vi "ReallyComplicatedSonar (SubVI).vi"(11 "Activate Shoot":bool) -> ()   [LabVIEW 2017]
uses:
  <vilib>/Rock Robotics/WPI/Solenoid/WPI_SolenoidValue.ctl
  <vilib>/Rock Robotics/WPI/Utilities/WPI_GetSetVariantRefNum.vi
  <vilib>/Rock Robotics/WPI/RobotDrive/WPI_RobotDriveArcadeDrive_Standard(NoSaturation).vi
  <vilib>/Rock Robotics/WPI/Solenoid/WPI_SolenoidSetEnum.vi
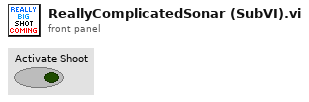
[diagram p1: front panel]
types:
  T1 = typedef "WPI_SolenoidValue.ctl" = enum16{"Off", "On", "Forward", "Reverse"}
  T2 = typedef "WPI_RobotDriveDevRef.ctl" = cluster{"DevStatus":errorcluster, "Motors[]":T3[], "Square Inputs":bool, "Max Output":dbl}
  T3 = typedef "WPI_MotorControlDeviceRef.ctl" = cluster{"DeviceStatus":errorcluster, "Type":T4, "PWM":cluster{"PWM Channel":T5, "DeadBand":T6}, "CAN":cluster{"Device Number":u8, "SetOutput VI Ref":variant, "GetOutput VI Ref":variant, "Enable VI Ref":variant, "Disable VI Ref":variant, "Data":variant}, "Invert":bool, "DIO PWM":cluster{"PWM \"Enable\" Channel":T5, "DIOChannel":T7, "PWM Rate":dbl}}
  T4 = typedef "WPI_MotorControlType.ctl" = enum16{"PWM", "CAN", "DIO PWM"}
  T5 = typedef "FPGA_DIOPWMChannel.ctl" = enum8{"PWM 0", "PWM 1", "PWM 2", "PWM 3", "PWM 4", "PWM 5", "PWM 6", "PWM 7", "PWM 8", "PWM 9", "PWM MXP 0", "PWM MXP 1", "PWM MXP 2", "PWM MXP 3", "PWM MXP 4", "PWM MXP 5", "PWM MXP 6", "PWM MXP 7", "PWM MXP 8", "PWM MXP 9", "Invalid"}
  T6 = typedef "WPI_PWMDeadband.ctl" = cluster{"Name":string, "maxPositivePwm":i32, "minPositivePwm":i32, "centerPwm":i32, "maxNegativePwm":i32, "minNegativePwm":i32, "angularRange":u16}
  T7 = typedef "FPGA_DIOChannel.ctl" = enum8{"DIO 0", "DIO 1", "DIO 2", "DIO 3", "DIO 4", "DIO 5", "DIO 6", "DIO 7", "DIO 8", "DIO 9", "DIO MXP 0", "DIO MXP 1", "DIO MXP 2", "DIO MXP 3", "DIO MXP 4", "DIO MXP 5", "DIO MXP 6", "DIO MXP 7", "DIO MXP 8", "DIO MXP 9", "DIO MXP 10", "DIO MXP 11", "DIO MXP 12", "DIO MXP 13", "DIO MXP 14", "DIO MXP 15", "SPI Port CS1", "SPI Port CS2", "SPI Port CS3", "SPI Port MISO", "SPI Port MOSI", "Invalid"}
  T8 = typedef "DriveMotors.ctl" = cluster{"MotorControlDevRef":T3, "MotorControlDevRef":T3, "MotorControlDevRef":T3, "MotorControlDevRef":T3, "MotorControlDevRef":T3, "MotorControlDevRef":T3}
  T9 = typedef "WPI_SolenoidDevRef.ctl" = cluster{"DevStatus":errorcluster, "Pneumatics Control Module":u8, "Forward Solenoid Channel":T10, "Reverse Solenoid Channel":T10}
  T10 = typedef "WPI_SolenoidChannel.ctl" = enum8{"Solenoid 0", "Solenoid 1", "Solenoid 2", "Solenoid 3", "Solenoid 4", "Solenoid 5", "Solenoid 6", "Solenoid 7", "Invalid"}
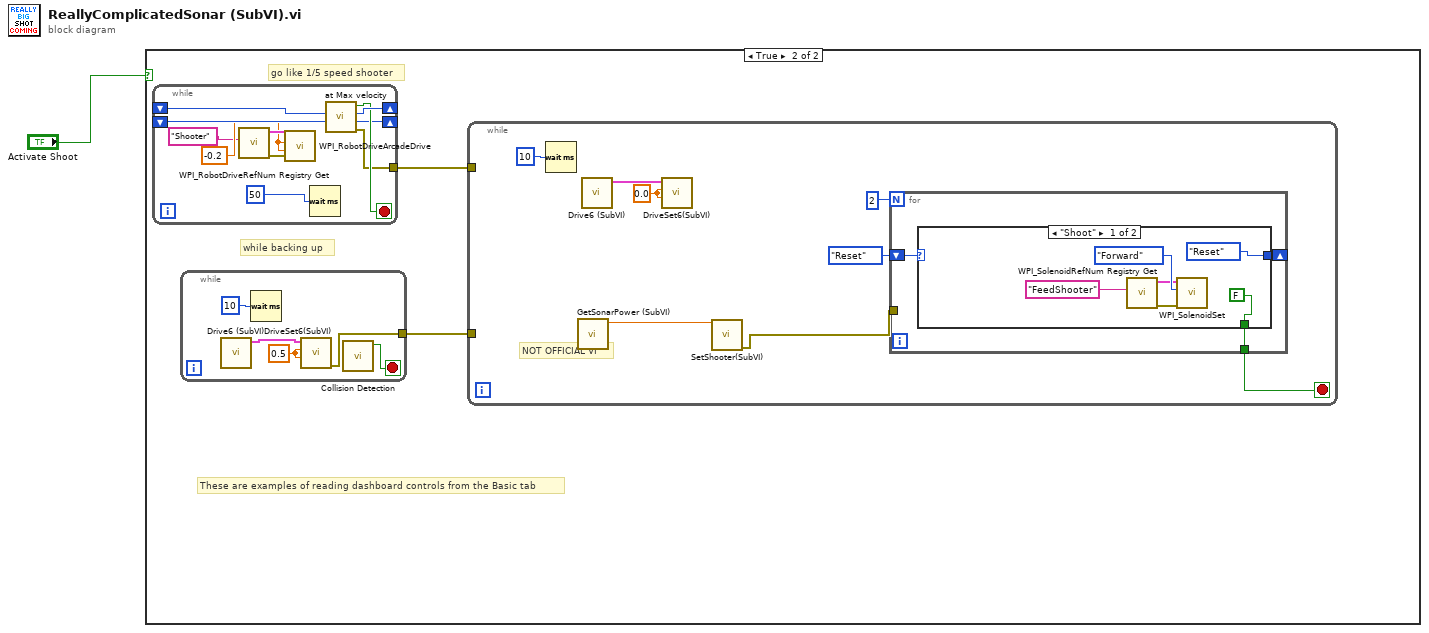
[diagram p0: block diagram]
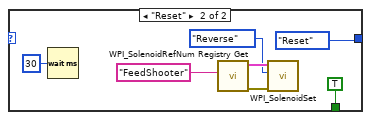
[diagram p3: hidden frame]
diagram:
  # "These are examples of reading dashboard controls from the Basic tab"
  n1 = case shown="True" "Activate Shoot" {
    frame False {
    }
    frame True {
      # "while backing up"
      # "go like 1/5 speed shooter"
      n2 = while {
        shift-right: [w40] -> _
        shift-left: _ -> [w42]
        shift-right: [w38] -> _
        shift-left: _ -> [w41]
        tunnel: [w37] -> w2
        stop <- w39 stop-if-true
        w34 = -0.2 ("Percentage")
        n3 = call <vilib>:"WPI_RobotDriveRefNum Registry Get.vi"("refnum name"="Shooter") -> ("error out"=w36:errorcluster, "RobotDriveDevRef"=w35:T2)  [unwired: 9 in]
        n4 = call-poly <vilib>:"WPI_RobotDriveArcadeDrive.vi"("error in (no error)"=w36, "Y axis value"=w34, "X axis value"=w34, "RobotDriveDevRef"=w35) -> ()  [unwired: 5 in, 3 out]
        n5 = Wait (ms)(milliseconds to wait=u32 50) -> ()  [unwired: 1 out]
        n6 = call "at Max velocity.vi"("Previous Velocity 2"=w41, "Previous Velocity"=w42) -> ("error out 2"=w37:errorcluster, "New Velocity 2"=w38:i32, "New Velocity"=w40:i32, "Max Velocity"=w39:bool)  [unwired: 6 in]
      }
      n7 = while {
        tunnel: [w28] -> w3
        stop <- w32 stop-if-true
        w29 = 0.5 ("Right")
        n8 = call "Drive6 (SubVI).vi"() -> ("DriveControlDevRef"=w30:T8)  [unwired: 10 in, 1 out]
        n9 = Wait (ms)(milliseconds to wait=u32 10) -> ()  [unwired: 1 out]
        n10 = call "DriveSet6(SubVI).vi"("Left"=w29, "Right"=w29, "output cluster"=w30) -> ("error out"=w28:errorcluster)  [unwired: 7 in, 1 out]
        n11 = call "Collision Detection.vi"() -> ("Colision Detected"=w32:bool)  [unwired: 11 in]
      }
      n12 = while {
        tunnel: w3 -> [_]
        tunnel: w2 -> [_]
        stop <- w5 stop-if-true
        w9 = 0.0 ("Right")
        # "NOT OFFICIAL VI"
        n13 = Wait (ms)(milliseconds to wait=u32 10) -> ()  [unwired: 1 out]
        n14 = call "GetSonarPower (SubVI).vi"() -> ("Value"=w8:dbl)  [unwired: 11 in]
        n15 = call "Drive6 (SubVI).vi"() -> ("DriveControlDevRef"=w10:T8)  [unwired: 10 in, 1 out]
        n16 = call "DriveSet6(SubVI).vi"("Left"=w9, "Right"=w9, "output cluster"=w10) -> ()  [unwired: 7 in, 2 out]
        n17 = call "SetShooter(SubVI).vi"("Velocity"=w8) -> ("error out"=w4:errorcluster)  [unwired: 10 in]
        n18 = for {
          N: 2 -> [_]
          shift-right: [w13] -> _
          shift-left: enum16{"Shoot", "Reset"}."Reset" -> [w14]
          tunnel: [w12] -> w5
          tunnel: w4 -> [_]
          n19 = case shown="\"Shoot\"" w14 {
            tunnel: [enum16{"Shoot", "Reset"}."Reset" enum16{"Shoot", "Reset"}."Reset"] -> w13
            tunnel: [FALSE TRUE] -> w12
            frame "Shoot" {
              n20 = call <vilib>:"WPI_SolenoidRefNum Registry Get.vi"("refnum name"="FeedShooter") -> ("error out"=w17:errorcluster, "SolenoidDevRef"=w18:T9)  [unwired: 9 in]
              n21 = call-poly <vilib>:"WPI_SolenoidSet.vi"("error in (no error)"=w17, "Value"=WPI_SolenoidValue."Forward", "SolenoidDevRef"=w18) -> ()  [unwired: 7 in, 2 out]
            }
            frame "Reset" {
              n22 = Wait (ms)(milliseconds to wait=u32 30) -> ()  [unwired: 1 out]
              n23 = call <vilib>:"WPI_SolenoidRefNum Registry Get.vi"("refnum name"="FeedShooter") -> ("error out"=w26:errorcluster, "SolenoidDevRef"=w27:T9)  [unwired: 9 in]
              n24 = call-poly <vilib>:"WPI_SolenoidSet.vi"("error in (no error)"=w26, "Value"=WPI_SolenoidValue."Reverse", "SolenoidDevRef"=w27) -> ()  [unwired: 7 in, 2 out]
            }
          }
        }
      }
    }
  }
